vi "Read Params from INI Section.vi"(8 "error in (no error)":errorcluster, 9 "Parameters In":variant, 10 "Refnum in":T2, 11 "Analyze q-Factor in":refnum<class "Analyze q-Factor.lvclass">) -> (0 "error out":errorcluster, 1 "Parameters Out":variant, 2 "Refnum out":T2, 3 "Analyze q-Factor out":refnum<class "Analyze q-Factor.lvclass">)   [LabVIEW 2020, in "Analyze.lvlib" / "Analyze q-Factor.lvclass"]
uses:
  Analyze q-Factor.lvclass
  <vilib>/Utility/config.llb/Config Data RefNum.ctl
  Width Method.ctl
  <vilib>/Utility/config.llb/Read Key (String).vi
  <vilib>/Utility/config.llb/NI_LVConfig.lvlib
panel:
  in  "Method":T1
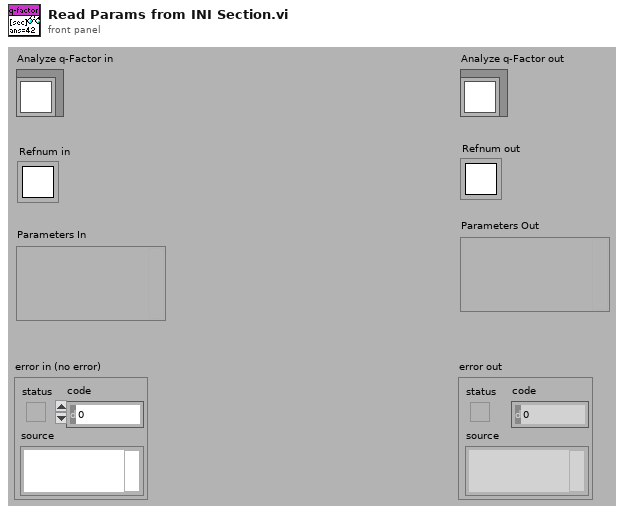
[diagram p1: front panel]
types:
  T1 = typedef "Width Method.ctl" = enum16{"FWHM", "1/e", "1/e^2", "80%", "90%"}
  T2 = typedef "NI_LVConfig.lvlib/Config Data RefNum.ctl" = refnum<k1>
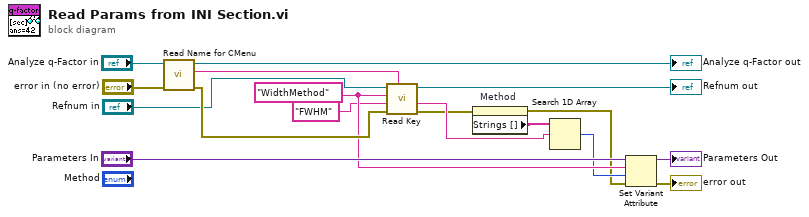
[diagram p0: block diagram]
diagram:
  w7 = "WidthMethod" ("name")
  n1 = call-dynamic "Read Name for CMenu.vi"("error in (no error)"="error in (no error)", "Analyze BaseClass in"="Analyze q-Factor in") -> ("error out"=w15:errorcluster, "Name for Context menu"=w14:string, "Analyze BaseClass out"=→"Analyze q-Factor out":refnum<class "Analyze q-Factor.lvclass">)  [unwired: 7 in]
  n2 = call-poly <vilib>:"Read Key.vi"("section"=w14, "error in (no error)"=w15, "default value"="FWHM" ("name"), "key"=w7, "refnum"="Refnum in") -> ("error out"=w2:errorcluster, "value"=w4:string, "refnum out"=→"Refnum out":T2)  [unwired: 3 in, 1 out]
  n3 = property on="Method" class="Enum (strict)"(error in=w2) -> (error out=w1:errorcluster, "Strings []"=w5:string[])  [unwired: 1 in, 1 out]
  n4 = Search 1D Array(1D array=w5, element=w4) -> (index of element=w3:i32)  [unwired: 1 in]
  n5 = Set Variant Attribute(Variant="Parameters In", name=w7, value=w3, error in=w1) -> (Variant out=→"Parameters Out":variant, error out=→"error out":errorcluster)  [unwired: 1 out]
